vi "scan.vi"(11 "NXT":T1) -> (0 "Array":i32[](array[numeric]), 3 "NXT 2":T1={"Hardware"="NXT", "Flattened String"=""} caption="NXT")   [LabVIEW 2012]
uses:
  <vilib>/NXT/Subs/LVHSConnector.ctl
  <vilib>/NXT/Subs/MotorOutput.ctl
  <vilib>/NXT/Dual Mode Library/Motors/MotorBrake.vi
  <vilib>/NXT/Dual Mode Library/Waits/Wait_Num(msec).vi
  <vilib>/NXT/Dual Mode Library/Waits/Wait_Num.vi
  <vilib>/NXT/Dual Mode Library/Display/drawText.vi
  <vilib>/NXT/Dual Mode Library/prims/reverseArray/reverseArray_float.vi
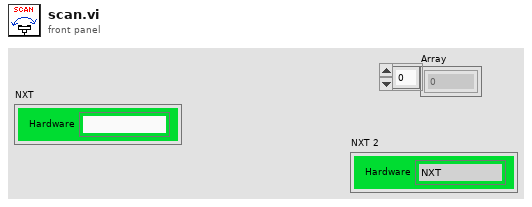
[diagram p1: front panel]
types:
  T1 = typedef "LVHSConnector.ctl" = cluster{"Hardware":string, "Flattened String":string}
  T2 = typedef "MotorOutput.ctl" = u8
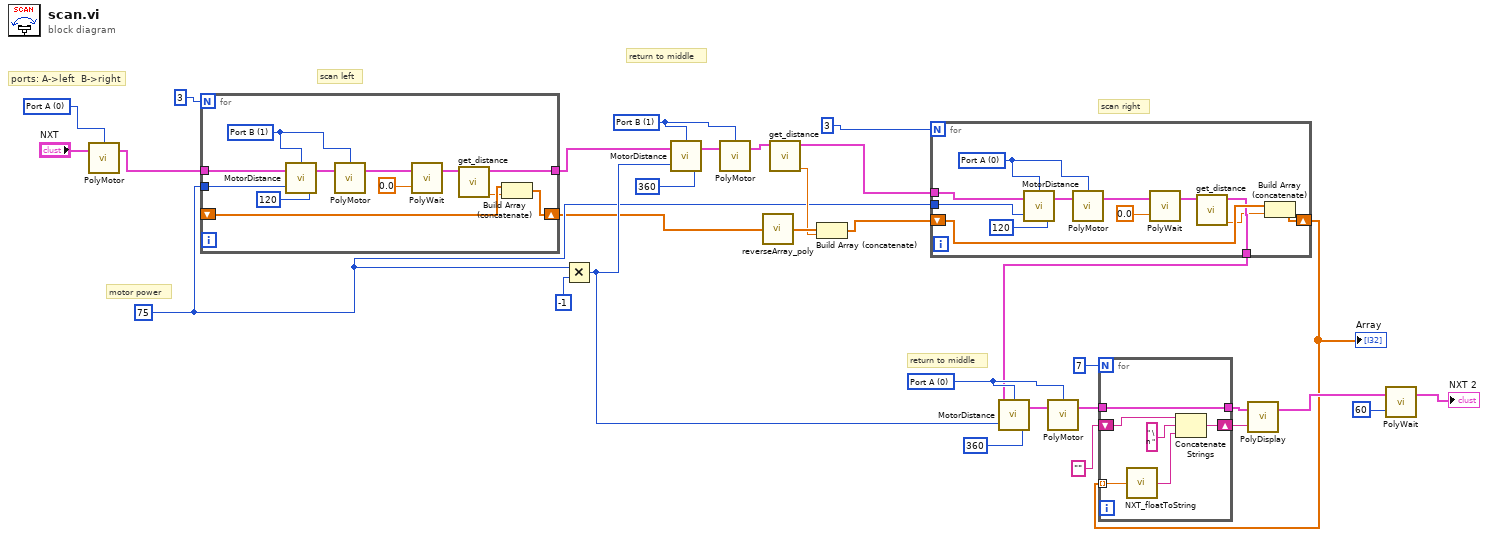
[diagram p0: block diagram]
diagram:
  w22 = T2 0 items=["Port A"=0, "Port B"=1, "Port C"=2, "Ports A & B"=4, "Ports A & C"=5, "Ports B & C"=6, "as"=3] ("Output Port (All Ports)")
  w2 = 75
  w23 = T2 1 items=["Port A"=0, "Port B"=1, "Port C"=2, "Ports A & B"=4, "Ports A & C"=5, "Ports B & C"=6, "as"=3] ("Output Port (All Ports)")
  w31 = T2 0 items=["Port A"=0, "Port B"=1, "Port C"=2, "Ports A & B"=4, "Ports A & C"=5, "Ports B & C"=6, "as"=3] ("Output Port (All Ports)")
  # "motor power"
  # "return to middle"
  # "scan right"
  # "return to middle"
  # "scan left"
  # "ports: A->left  B->right"
  n1 = call-poly <vilib>:"PolyMotor.vi"("NXT"="NXT", "Port (All Ports)"=w31) -> ("NXT"=w26:T1)  [unwired: 2 in]
  n2 = for {
    N: 3 -> [_]
    tunnel: w26 -> [w43]
    tunnel: w2 -> [w42]
    tunnel: [w33] -> w27
    shift-right: [w35] -> w1
    shift-left: _ -> [w36]
    w41 = T2 1 items=["Port A"=0, "Port B"=1, "Port C"=2, "Ports A & B"=4, "Ports A & C"=5, "Ports B & C"=6, "as"=3] ("Output Port (All Ports)")
    n3 = call <vilib>:"MotorDistance.vi"("Power (75)"=w42, "Angle of Rotation (360)"=120, "NXT"=w43, "Output Port (All Ports)"=w41) -> ("NXT"=w39:T1)
    n4 = call-poly <vilib>:"PolyMotor.vi"("NXT"=w39, "Port (All Ports)"=w41) -> ("NXT"=w38:T1)  [unwired: 2 in]
    n5 = call-poly <vilib>:"PolyWait.vi"("Time (100 msec)"=sgl 0.0 ("Time (1 sec)"), "NXT"=w38) -> ("NXT"=w34:T1)  [unwired: 2 in]
    n6 = call "get_distance.vi"("NXT"=w34) -> ("Distance (cm)"=w32:dbl, "NXT 2"=w33:T1)  [unwired: 9 in]
    n7 = Build Array (concatenate)(w36, w32) -> (w35:dbl[])
  }
  n8 = Multiply(x=w2, y=-1) -> (x*y=w19:i32)
  n9 = call <vilib>:"MotorDistance.vi"("Power (75)"=w19, "Angle of Rotation (360)"=360, "NXT"=w27, "Output Port (All Ports)"=w23) -> ("NXT"=w24:T1)
  n10 = call-poly <vilib>:"PolyMotor.vi"("NXT"=w24, "Port (All Ports)"=w23) -> ("NXT"=w11:T1)  [unwired: 2 in]
  n11 = call-poly <vilib>:"reverseArray_poly.vi"("array"=w1) -> ("reversed array"=w9:dbl[])
  n12 = call "get_distance.vi"("NXT"=w11) -> ("Distance (cm)"=w8:dbl, "NXT 2"=w10:T1)  [unwired: 9 in]
  n13 = Build Array (concatenate)(w9, w8) -> (w7:dbl[])
  n14 = for {
    N: 3 -> [_]
    tunnel: w10 -> [w51]
    tunnel: w2 -> [w52]
    shift-right: [w47] -> w5
    shift-left: w7 -> [w48]
    tunnel: [w45] -> w3
    w54 = T2 0 items=["Port A"=0, "Port B"=1, "Port C"=2, "Ports A & B"=4, "Ports A & C"=5, "Ports B & C"=6, "as"=3] ("Output Port (All Ports)")
    n15 = call <vilib>:"MotorDistance.vi"("Power (75)"=w52, "Angle of Rotation (360)"=120, "NXT"=w51, "Output Port (All Ports)"=w54) -> ("NXT"=w53:T1)
    n16 = call-poly <vilib>:"PolyMotor.vi"("NXT"=w53, "Port (All Ports)"=w54) -> ("NXT"=w49:T1)  [unwired: 2 in]
    n17 = call-poly <vilib>:"PolyWait.vi"("Time (100 msec)"=sgl 0.0 ("Time (1 sec)"), "NXT"=w49) -> ("NXT"=w46:T1)  [unwired: 2 in]
    n18 = call "get_distance.vi"("NXT"=w46) -> ("Distance (cm)"=w44:dbl, "NXT 2"=w45:T1)  [unwired: 9 in]
    n19 = Build Array (concatenate)(w48, w44) -> (w47:dbl[])
  }
  "Array" <- w5
  n20 = call <vilib>:"MotorDistance.vi"("Power (75)"=w19, "Angle of Rotation (360)"=360, "NXT"=w3, "Output Port (All Ports)"=w22) -> ("NXT"=w21:T1)
  n21 = call-poly <vilib>:"PolyMotor.vi"("NXT"=w21, "Port (All Ports)"=w22) -> ("NXT"=w18:T1)  [unwired: 2 in]
  n22 = for {
    N: 7 -> [_]
    tunnel: w18 -> [w58]
    tunnel: [w58] -> w14
    shift-right: [w59] -> w13
    shift-left: "" ("Text") -> [w61]
    tunnel: w5 -> [w57] mode=indexing
    n23 = call <vilib>:"NXT_floatToString.vi"("number"=w57) -> ("string"=w60:string)
    n24 = Concatenate Strings(w61, " \n " ("Text"), w60) -> (w59:string)
  }
  n25 = call-poly <vilib>:"PolyDisplay.vi"("Text"=w13, "NXT"=w14) -> ("NXT"=w12:T1)  [unwired: 2 in]
  n26 = call-poly <vilib>:"PolyWait.vi"("Time (1 sec)"=60, "NXT"=w12) -> ("NXT"=→"NXT 2":T1)  [unwired: 2 in]
